vi "Update Plot.vi"(7 "Buffer":bool, 8 "Source Voltage":dbl, 9 "XY Graphs":refnum<vi>[](array[refnum]), 10 "Source Voltage[]":dbl[](array[numeric]), 11 "Plot colors":u32[](array[numeric])) -> ()   [LabVIEW 2021, in "PMIC UI.lvlib"]
uses:
  PMIC UI.lvlib
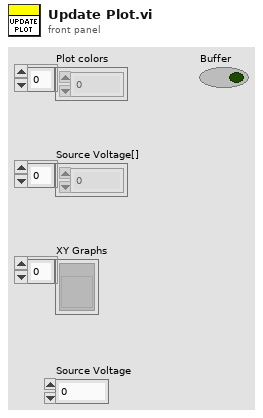
[diagram p1: front panel]
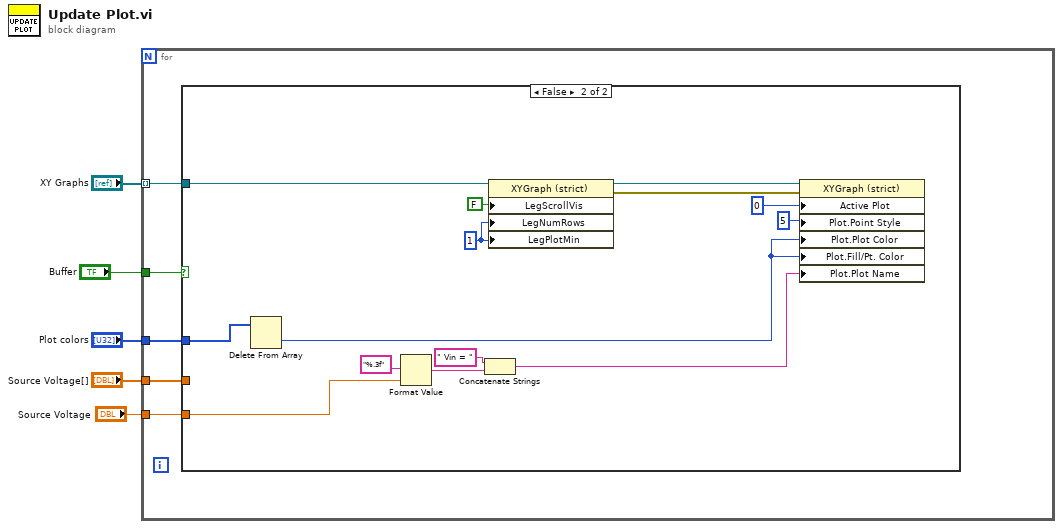
[diagram p0: block diagram]
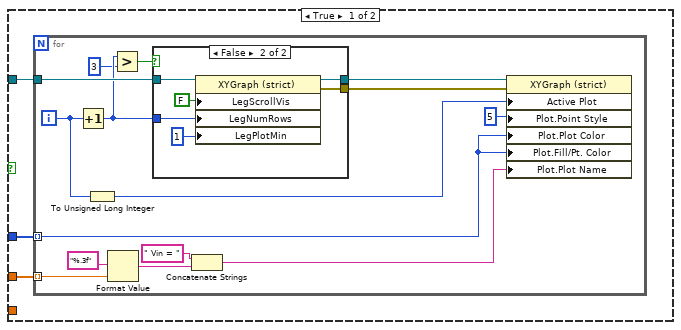
[diagram p2: hidden frame]
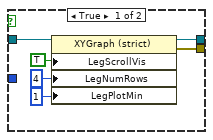
[diagram p3: hidden frame]
diagram:
  n1 = for {
    tunnel: "Source Voltage[]" -> [w10]
    tunnel: "XY Graphs" -> [w9] mode=indexing
    tunnel: "Plot colors" -> [w8]
    tunnel: "Buffer" -> [w7]
    tunnel: "Source Voltage" -> [w6]
    n2 = case shown="False" w7 {
      tunnel: w10 -> [w13 _]
      tunnel: w9 -> [w12 w54]
      tunnel: w8 -> [w11 w53]
      tunnel: w6 -> [_ w41]
      frame True {
        n3 = for {
          tunnel: w13 -> [w25] mode=indexing
          tunnel: w12 -> [w20]
          tunnel: w11 -> [w23] mode=indexing
          i -> [w21]
          n4 = Increment(x=w21) -> (x+1=w16:i32)
          n5 = To Unsigned Long Integer(number=w21) -> (unsigned 32bit integer=w24:u32)
          n6 = Format Value(format string="%.3f", value (0)=w25) -> (output string=w28:string)  [unwired: 1 out]
          n7 = Greater?(x=w16, y=3 ("x")) -> (0:w14:bool)
          n8 = case shown="False" w14 {
            tunnel: w20 -> [w34 w40]
            tunnel: [w33 w39] -> w19
            tunnel: [w32 w38] -> w18
            tunnel: w16 -> [_ w35]
            frame True {
              n9 = property on="Property Node" class="XYGraph (strict)"(reference=w34, "LegScrollVis"=TRUE ("Legend:Scrollbar Visible"), "LegNumRows"=u32 4 ("Legend:Number of Rows"), "LegPlotMin"=1 ("y")) -> (reference out=w33:refnum<vi>, error out=w32:errorcluster)  [unwired: 1 in]
            }
            frame False {
              n10 = property on="Property Node" class="XYGraph (strict)"(reference=w40, "LegScrollVis"=FALSE ("Legend:Scrollbar Visible"), "LegNumRows"=w35, "LegPlotMin"=1 ("y")) -> (reference out=w39:refnum<vi>, error out=w38:errorcluster)  [unwired: 1 in]
            }
          }
          n11 = Concatenate Strings(" Vin = " ("string"), w28) -> (w17:string)
          n12 = property on="Property Node" class="XYGraph (strict)"(reference=w19, error in=w18, "Active Plot"=w24, "Plot.Point Style"=u8 5, "Plot.Plot Color"=w23, "Plot.Fill/Pt. Color"=w23, "Plot.Plot Name"=w17) -> ()  [unwired: 2 out]
        }
      }
      frame False {
        w42 = 1 ("y")
        n13 = Delete From Array(array=w53) -> (deleted portion=w52:u32)  [unwired: 2 in, 1 out]
        n14 = Format Value(format string="%.3f", value (0)=w41) -> (output string=w51:string)  [unwired: 1 out]
        n15 = Concatenate Strings(" Vin = " ("string"), w51) -> (w44:string)
        n16 = property on="Property Node" class="XYGraph (strict)"(reference=w54, "LegScrollVis"=FALSE ("Legend:Scrollbar Visible"), "LegNumRows"=w42, "LegPlotMin"=w42) -> (reference out=w46:refnum<vi>, error out=w45:errorcluster)  [unwired: 1 in]
        n17 = property on="Property Node" class="XYGraph (strict)"(reference=w46, error in=w45, "Active Plot"=0 ("number"), "Plot.Point Style"=u8 5, "Plot.Plot Color"=w52, "Plot.Fill/Pt. Color"=w52, "Plot.Plot Name"=w44) -> ()  [unwired: 2 out]
      }
    }
  }
